vi "Configure PMU.vi"(8 "error in (no error)":errorcluster, 11 "Phasor Measurement Unit in":refnum<class "Phasor Measurement Unit.lvclass">) -> (0 "error out":errorcluster, 3 "Phasor Measurement Unit out":refnum<class "Phasor Measurement Unit.lvclass">)   [LabVIEW 2018, in "S3DK.lvlib" / "PMU Recorder Light.lvlib" / "Phasor Measurement Unit.lvclass"]
uses:
  Phasor Measurement Unit.lvclass
  Phasor Measurement Unit.lvclass/Phasor Measurement Unit.ctl
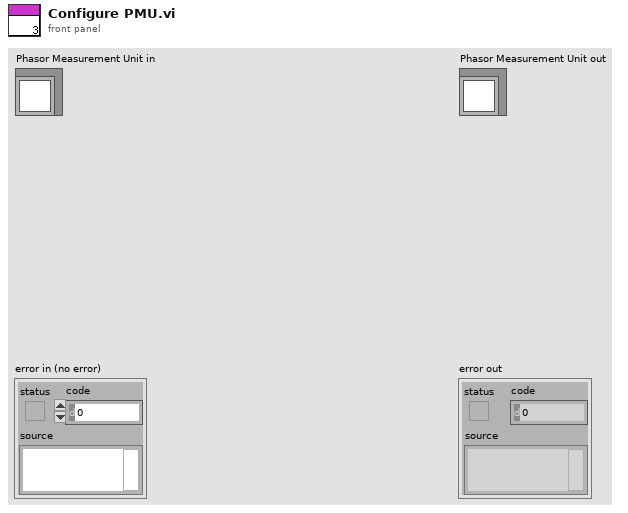
[diagram p1: front panel]
types:
  T1 = cluster{"PMU Configuration ":cluster{"PMU ID Code":i32, "PMU Name":string, "Nominal Frequency":sgl, "Format Code":i32, "Configuration Change Count":i32, "Number of Phasors":i32, "Number of Analog":i32, "Number of Digital":i32, "Status":bool}, "Phasor Configuration":cluster{"Group Name":string, "Channel Name":string, "Channel Name Real":string, "Channel Name Imaginary":string, "Group Index":i32, "Channel Index":i32, "isValid?":bool, "Scaling":sgl, "Type":i32}[], "Analog Configuration":cluster{"Group Name":string, "Channel Name":string, "Group Index":i32, "Channel Index":i32, "isValid?":bool, "Scaling":sgl, "Type":i32}[], "Digital Configuration":cluster{"Group Name":string, "Channel Name":string, "Group Index":i32, "Channel Index":i32, "isValid?":bool, "Type":i32}[]}
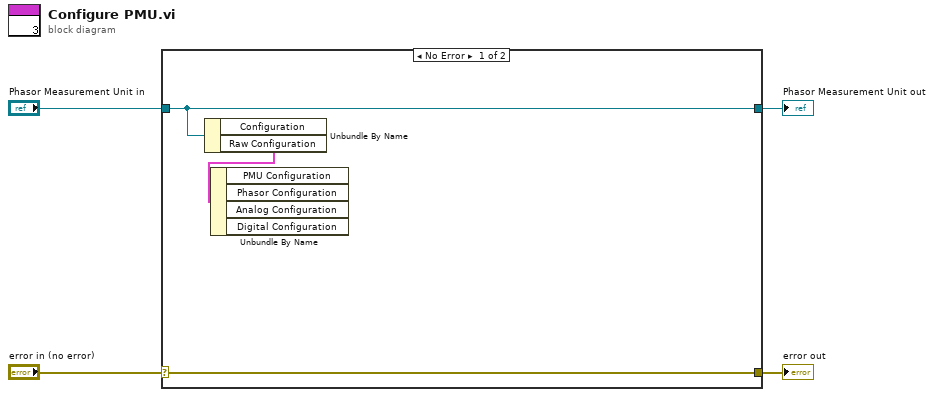
[diagram p0: block diagram]
diagram:
  n1 = case shown="No Error" "error in (no error)" {
    selector: "error in (no error)" -> [w7 w9]
    tunnel: [w7 w9] -> w3
    tunnel: [w6 w8] -> w1
    tunnel: "Phasor Measurement Unit in" -> [w6 w8]
    frame No Error {
      n2 = Unbundle By Name(w6) -> ("Raw Configuration"=w5:T1)  [unwired: 1 out]
      n3 = Unbundle By Name(w5) -> ()  [unwired: 4 out]
    }
    frame Error {
    }
  }
  "error out" <- w3
  "Phasor Measurement Unit out" <- w1
